vi "Initialize Accel Task.vi"(8 "error in (no error)":errorcluster, 9 "Accel TDMS File":refnum<k34>, 10 "Accel Rate":i32, 11 "Accelerometer in":refnum<class "Accelerometer.lvclass">) -> (0 "error out":errorcluster, 3 "Accelerometer out":refnum<class "Accelerometer.lvclass">)   [LabVIEW 2020, in "Accelerometer.lvlib" / "Accelerometer.lvclass"]
uses:
  Accelerometer.lvclass
  C:/Program Files/National Instruments/LabVIEW 2020/vi.lib/ActorFramework/Actor/Actor.lvclass
  <vilib>/ActorFramework/Actor/Actor.lvclass/Actor.ctl
  <vilib>/ActorFramework/Message Enqueuer/Message Enqueuer.lvclass/Message Enqueuer.ctl
  Accelerometer.lvclass/Accelerometer.ctl
  <vilib>/ActorFramework/Message Enqueuer/Init from Existing Queue.vi
  <vilib>/ActorFramework/Message Enqueuer/Enqueue.vi
  <vilib>/ActorFramework/Stop Msg/Stop Msg.lvclass
  C:/Program Files/National Instruments/LabVIEW 2020/vi.lib/ActorFramework/Message/Message.lvclass
  <instrlib>/Phidgets/Phidget Accelerometer/Public/AccelerometerStart.vi
  <vilib>/ActorFramework/Message Priority Queue/Priority Enqueue.vi
  <vilib>/ActorFramework/Message Enqueuer/Message Enqueuer.lvclass
  <vilib>/ActorFramework/Actor/Actor.lvclass
  <instrlib>/Phidgets/Phidget Common/Phidget Common.lvlib
  <instrlib>/Phidgets/Phidget Accelerometer/Phidget Accelerometer.lvlib
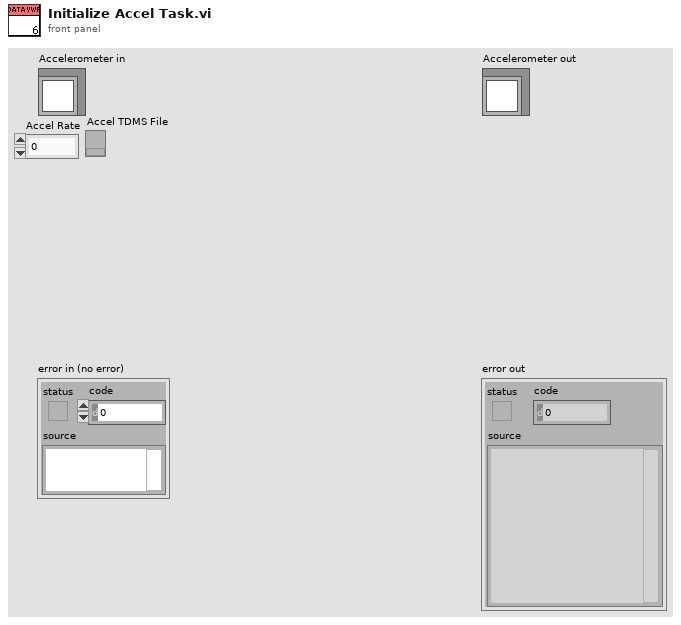
[diagram p1: front panel]
types:
  T1 = cluster{"Serial Number":i32, "Channel":i32, "Port":i32}
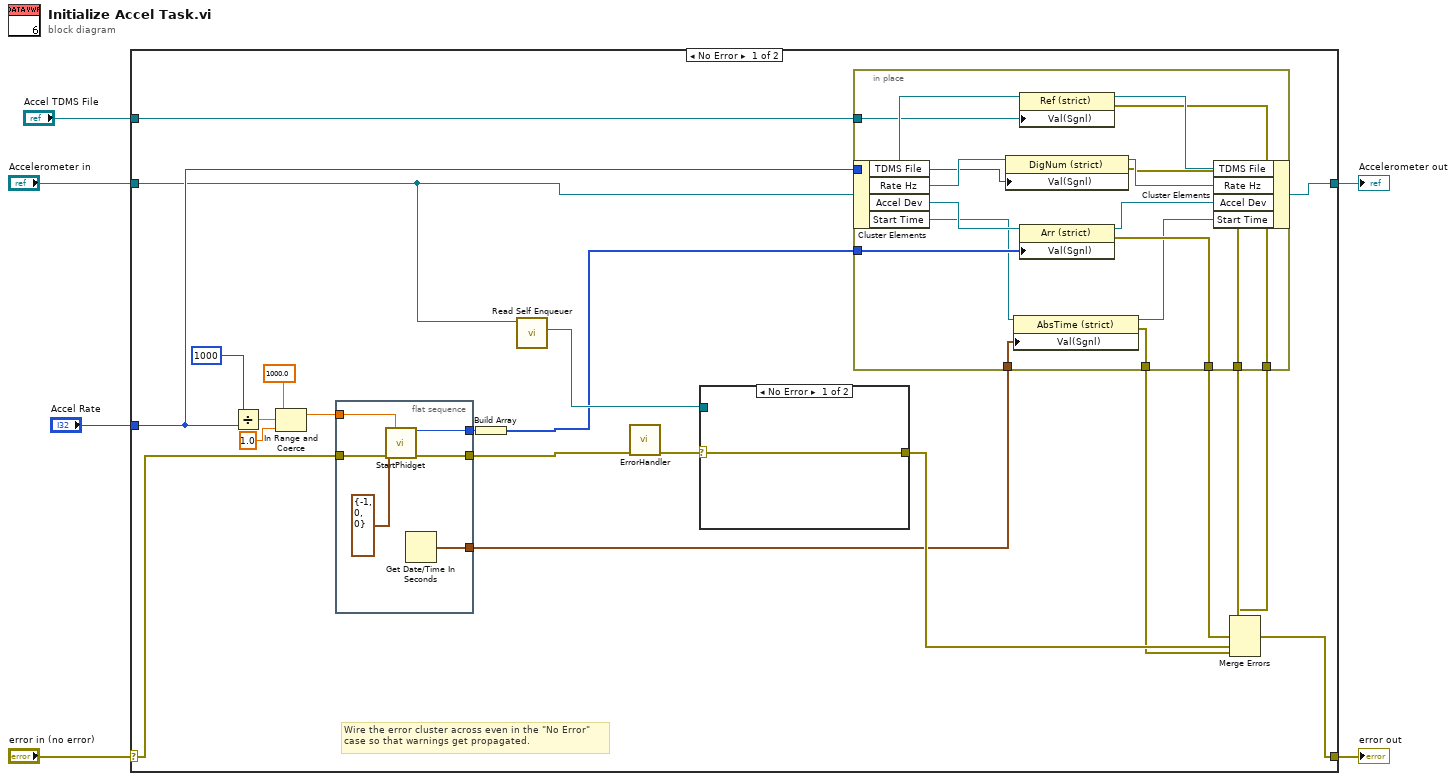
[diagram p0: block diagram]
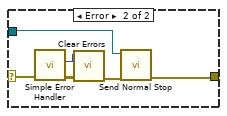
[diagram p2: hidden frame]
diagram:
  n1 = case shown="No Error" "error in (no error)" {
    selector: "error in (no error)" -> [w19 w59]
    tunnel: [w16 w59] -> w5
    tunnel: [w22 w58] -> w3
    tunnel: "Accelerometer in" -> [w20 w58]
    tunnel: "Accel Rate" -> [w21 _]
    tunnel: "Accel TDMS File" -> [w15 _]
    frame No Error {
      # "Wire the error cluster across even in the \"No Error\"\ncase so that warnings get propagated."
      n2 = Divide(x=1000, y=w21) -> (x/y=w26:dbl)
      n3 = In Range and Coerce(upper limit=1000.0, x=w26, lower limit=1.0) -> (coerced(x)=w9:dbl)  [unwired: 1 out]
      n4 = flat-sequence {
        tunnel: [w34] -> w28
        tunnel: w19 -> [w32]
        tunnel: [w31] -> w10
        tunnel: w9 -> [w30]
        tunnel: [w29] -> w8
        frame #0 {
          n5 = call-poly <instrlib>:"StartPhidget.vi"("Device Info"=T1 {"Serial Number"=-1, "Channel"=0, "Port"=0}, "Data Interval"=w30, "error in (no error)"=w32) -> ("Phidget ID"=w34:u64, "error out"=w31:errorcluster)  [unwired: 9 in, 2 out]
          n6 = Get Date/Time In Seconds() -> (seconds since 1Jan1904=w29:timestamp)
        }
      }
      n7 = Build Array(w28) -> (w11:u64[])
      n8 = call <vilib>:"Read Self Enqueuer.vi"("Actor"=w20) -> ("Self Enqueuer"=w23:refnum<class "Message Enqueuer.lvclass">)  [unwired: 10 in]
      n9 = call <instrlib>:"ErrorHandler.vi"("error in"=w10) -> ("error out"=w14:errorcluster)  [unwired: 9 in, 1 out]
      n10 = case shown="No Error" w14 {
        selector: w14 -> [w51 w57]
        tunnel: [w51 w52] -> w13
        tunnel: w23 -> [_ w53]
        frame No Error {
        }
        frame Error {
          n11 = call <vilib>:"Simple Error Handler.vi"("error in (no error)"=w57) -> ("code out"=w55:i32, "error out"=w56:errorcluster)  [unwired: 4 in, 3 out]
          n12 = call <vilib>:"Clear Errors.vi"("error in (no error)"=w56, "specific error code to clear (0: all)"=w55) -> ("error out"=w54:errorcluster)  [unwired: 4 in, 1 out]
          n13 = call <vilib>:"Send Normal Stop.vi"("error in (no error)"=w54, "Message Enqueuer"=w53) -> ("error out"=w52:errorcluster)  [unwired: 9 in]
        }
      }
      n14 = in-place {
        in-place-border: w11 -> [w46]
        in-place-border: w21 -> [w45]
        in-place-border: [w44] -> w18
        in-place-border: [w43] -> w17
        in-place-border: w15 -> [w40]
        in-place-border: [w39] -> w12
        in-place-border: w8 -> [w36]
        in-place-border: [w35] -> w7
        n15 = in-place-cluster #1(w20) -> ("TDMS File"=w42:refnum<vi>, "Rate Hz"=w50:refnum<vi>, "Accel Dev"=w48:refnum<vi>, "Start Time"=w38:refnum<vi>)
        n16 = property class="DigNum (strict)"(reference=w50, "Val(Sgnl)"=w45) -> (reference out=w49:refnum<vi>, error out=w43:errorcluster)  [unwired: 1 in]
        n17 = property class="AbsTime (strict)"(reference=w38, "Val(Sgnl)"=w36) -> (reference out=w37:refnum<vi>, error out=w35:errorcluster)  [unwired: 1 in]
        n18 = property class="Ref (strict)"(reference=w42, "Val(Sgnl)"=w40) -> (reference out=w41:refnum<vi>, error out=w39:errorcluster)  [unwired: 1 in]
        n19 = property class="Arr (strict)"(reference=w48, "Val(Sgnl)"=w46) -> (reference out=w47:refnum<vi>, error out=w44:errorcluster)  [unwired: 1 in]
        n20 = in-place-cluster #1("TDMS File"=w41, "Rate Hz"=w49, "Accel Dev"=w47, "Start Time"=w37) -> (w22:refnum<class "Accelerometer.lvclass">)
      }
      n21 = Merge Errors(w12, w17, w18, w13, w7) -> (w16:errorcluster)
    }
    frame Error {
    }
  }
  "error out" <- w5
  "Accelerometer out" <- w3
